vi "AI_InstantAI v1.vi"() -> ()   [LabVIEW 2013]
uses:
  <vilib>/Platform/TimedLoop/XDataNode/timing_clust.ctl
  <vilib>/Platform/TimedLoop/XDataNode/nitl_modes.ctl
  <vilib>/Platform/TimedLoop/XDataNode/wakeup.ctl
  <vilib>/platform/TimedLoop/XDataNode/XDataNode.xnode
  <vilib>/Platform/TimedLoop/XDataNode/XDNodeRunTimeDep.lvlib
panel:
  out "Array 2":dbl[][](array[numeric])
  out "loops":bool
  out "Waveform Graph":dbl[][](graph)
  in  "stop":bool
  out "error out":errorcluster
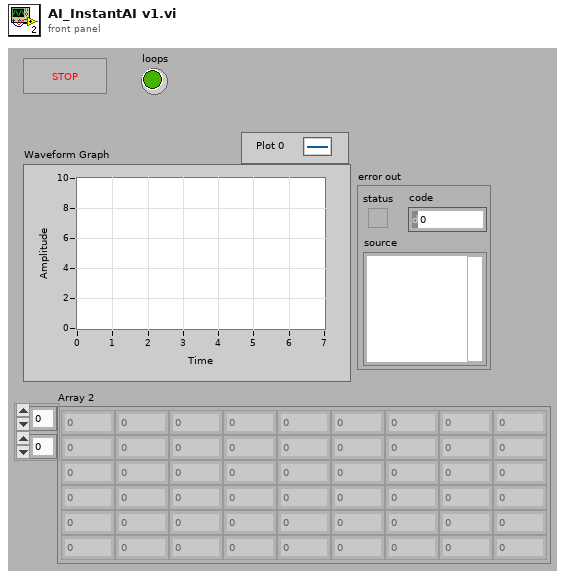
[diagram p1: front panel]
types:
  T1 = typedef "XDNodeRunTimeDep.lvlib/timing_clust.ctl" = cluster{"Expected End [f-1]":u64, "Actual End [f-1]":u64, "Finished Late? [f-1]":bool, "Expected End [i-1]":u64, "Actual End [i-1]":u64, "Finished Late? [i-1]":bool, "Expected Start [i]":u64, "Actual Start [i]":u64, "Expected Start [f]":u64, "Actual Start [f]":u64, "Source Name":string, "Structure Name":string, "Period":i64, "Deadline":i64, "Offset":i64, "Start":i64, "Priority":i32, "Timeout":i32, "Mode":T2, "Wakeup Reason":T3, "Error":errorcluster, "Source Type":string, "Secondary Source Type":string, "Global End Time":u64, "Global Start Time":u64, "Frame Duration":u64, "Iteration Duration":u64, "Assigned CPU":i32, "I/O Scan Engine Mode":u32}
  T2 = typedef "XDNodeRunTimeDep.lvlib/nitl_modes.ctl" = enum32{"No Change", "Process missed periods, maintain original phase", "Discard missed periods, maintain original phase", "Process missed periods, ignore original phase", "Discard missed periods, ignore original phase"}
  T3 = typedef "XDNodeRunTimeDep.lvlib/wakeup.ctl" = enum32{"Normal", "Aborted", "Asynchronous wakeup", "Timing source error", "Timed loop error", "Timeout"}
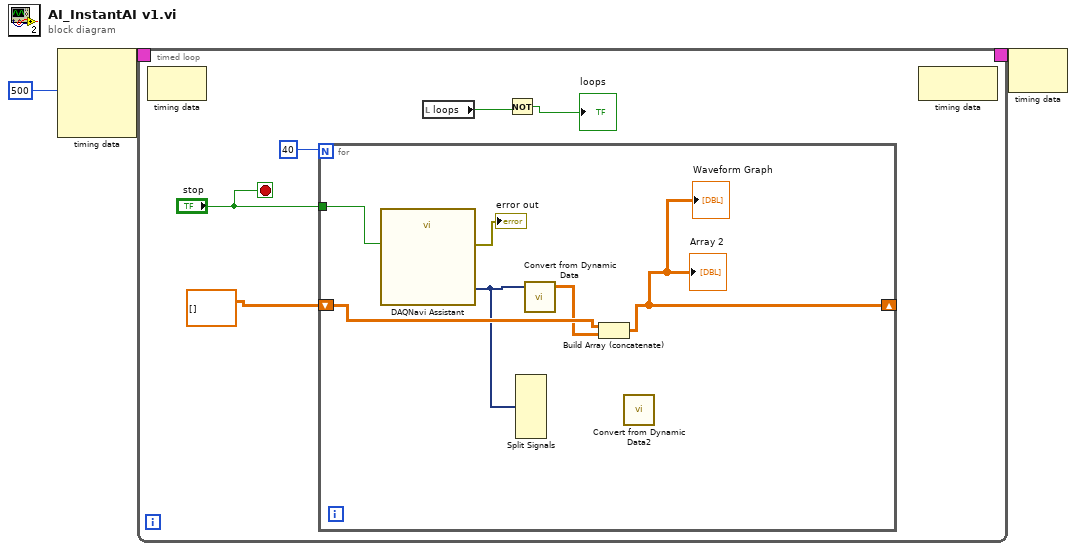
[diagram p0: block diagram]
diagram:
  n1 = node-c288(500) -> (w3:T1)  [unwired: 3 in]
  n2 = timed-loop {
    timing: w3 -> [_]
    timing-out: [_] -> w2
    stop <- "stop" stop-if-true
    n3 = node-c288() -> ()  [unwired: 1 in, 1 out]
    n4 = for {
      N: 40 -> [_]
      tunnel: "stop" -> [w15]
      shift-right: [w12] -> _
      shift-left: dbl[][] [] -> [w14]
      n5 = call "DAQNavi Assistant"("stop(true)"=w15) -> ("error out"=→"error out":errorcluster, "data out(DDT)"=w11:dynamicdata)  [unwired: 1 in, 16 out]
      n6 = Split Signals(w11) -> ()  [unwired: 8 in, 8 out]
      n7 = call "Convert from Dynamic Data"("Dynamic Data Type"=w11) -> ("Array"=w13:dbl[][])  [unwired: 3 in]
      n8 = Build Array (concatenate)(w14, w13) -> (w12:dbl[][])
      "Waveform Graph" <- w12
      "Array 2" <- w12
      n9 = call "Convert from Dynamic Data2"() -> ()  [unwired: 4 in, 1 out]
    }
    n10 = local read "loops"() -> (w6:bool)
    n11 = Not(x=w6) -> (.not. x?=→"loops":bool)
    n12 = node-c288() -> ()  [unwired: 1 in, 1 out]
  }
  n13 = node-c288(w2) -> ()  [unwired: 1 out]
